vi "FABR-Init Level Series.vi"(0 "Stimulus":T2={"Destination"="", "Rep rate (/sec)"=30.0, "Alternate Polarity"=FALSE, "Duration (ms)"=0.0, "Ramp (ms)"=16.0, "Fs (Hz)"=5.0, "Frame size (s)"=0.0}, 1 "Data Folder":path, 5 "Runtime In":T3, 7 "SCL in":T1[](array[typedef]), 11 "error in (no error)":errorcluster) -> (4 "Stimulus thru":T2={"Destination"="", "Rep rate (/sec)"=30.0, "Alternate Polarity"=FALSE, "Duration (ms)"=0.0, "Ramp (ms)"=16.0, "Fs (Hz)"=5.0, "Frame size (s)"=0.0}, 6 "Runtime Out":T3, 8 "SCL out":T1[](array[typedef]), 15 "error out":errorcluster)   [LabVIEW 2020]
uses:
  Utility VIs/Type Defs/Speaker ring.ctl
  Typedefs/FABR-Stimulus.ctl
  Typedefs/FABR-Runtime Data.ctl
  Typedefs/FABR-Stimulus Condition.ctl
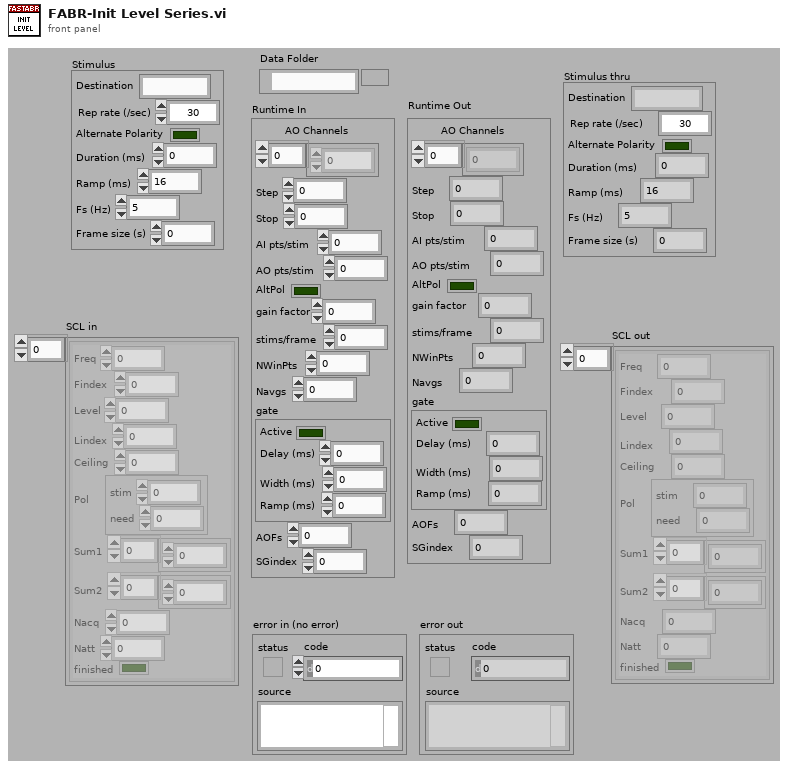
[diagram p1: front panel]
types:
  T1 = typedef "FABR-Stimulus Condition.ctl" = cluster{"Freq":dbl, "Findex":i32, "Level":dbl, "Lindex":i32, "Ceiling":dbl, "Pol":cluster{"stim":i32, "need":i32}, "Sum1":dbl[], "Sum2":dbl[], "Nacq":i32, "Natt":i32, "finished":bool}
  T2 = typedef "FABR-Stimulus.ctl" = cluster{"Destination":string, "Rep rate (/sec)":dbl, "Alternate Polarity":bool, "Duration (ms)":dbl, "Ramp (ms)":dbl, "Fs (Hz)":dbl, "Frame size (s)":dbl}
  T3 = typedef "FABR-Runtime Data.ctl" = cluster{"AO Channels":i32[], "Step":dbl, "Stop":i32, "AI pts/stim":i32, "AO pts/stim":i32, "AltPol":bool, "gain factor":dbl, "stims/frame":i32, "NWinPts":i32, "Navgs":i32, "gate":cluster{"Active":bool, "Delay (ms)":dbl, "Width (ms)":dbl, "Ramp (ms)":dbl}, "AOFs":dbl, "SGindex":i32}
  T4 = typedef "Speaker ring.ctl" = enum16{"Right primary", "Right secondary", "Left primary", "Left secondary"}
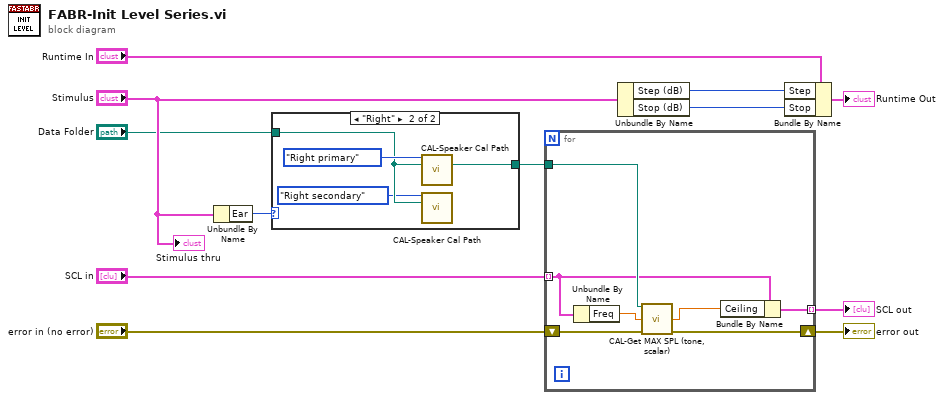
[diagram p0: block diagram]
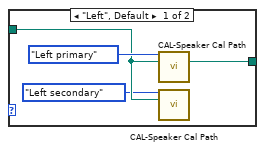
[diagram p2: hidden frame]
diagram:
  n1 = Unbundle By Name("Stimulus") -> ("Ear"=w10:enum16{"Right", "Left"})
  n2 = case shown="\"Right\"" w10 {
    tunnel: "Data Folder" -> [w15 w19]
    tunnel: [w13 w17] -> w4
    frame "Left", Default {
      n3 = call "CAL-Speaker Cal Path.vi"("Speaker"=Speaker_ring."Left primary", "Data Folder"=w15) -> ("Cal Path"=w13:path)  [unwired: 12 in, 1 out]
      n4 = call "CAL-Speaker Cal Path.vi"("Speaker"=Speaker_ring."Left secondary", "Data Folder"=w15) -> ()  [unwired: 12 in, 2 out]
    }
    frame "Right" {
      n5 = call "CAL-Speaker Cal Path.vi"("Speaker"=Speaker_ring."Right primary", "Data Folder"=w19) -> ("Cal Path"=w17:path)  [unwired: 12 in, 1 out]
      n6 = call "CAL-Speaker Cal Path.vi"("Speaker"=Speaker_ring."Right secondary", "Data Folder"=w19) -> ()  [unwired: 12 in, 2 out]
    }
  }
  n7 = for {
    tunnel: w4 -> [w25]
    shift-right: [w26] -> w9
    shift-left: "error in (no error)" -> [w27]
    tunnel: "SCL in" -> [w23] mode=indexing
    tunnel: [w21] -> w1 mode=indexing
    n8 = Unbundle By Name(w23) -> ("Freq"=w24:dbl)
    n9 = call "CAL-Get MAX SPL (tone, scalar).vi"("Cal Path"=w25, "Frequency (kHz)"=w24, "error in (no error)"=w27) -> ("Max SPL"=w22:dbl, "error out"=w26:errorcluster)  [unwired: 11 in]
    n10 = Bundle By Name(cluster=w23, "Ceiling"=w22) -> (w21:T1)
  }
  "error out" <- w9
  "SCL out" <- w1
  n11 = Unbundle By Name("Stimulus") -> ("Step (dB)"=w7:i32, "Stop (dB)"=w3:i32)
  n12 = Bundle By Name(cluster="Runtime In", "Step"=w7, "Stop"=w3) -> (→"Runtime Out":T3)
  "Stimulus thru" <- "Stimulus"
